vi "Field Mapper.vi"(9 "bandwidth":enum16{"20MHz", "40MHz", "80MHz"}(ring), 10 "subcarrier timing":T2={"subcarrier index"=0, "OFDM symbol index"=0, "frequency offset index"=0.0, "OFDM symbol start"=TRUE, "valid"=TRUE}, 11 "format":enum16{"NON_HT_OFDM", "VHT", "NON_HT_DUP_OFDM"}(ring)) -> (1 "field map":T1, 2 "subcarrier index":fxp<+/-,9,9>)   [LabVIEW 2020]
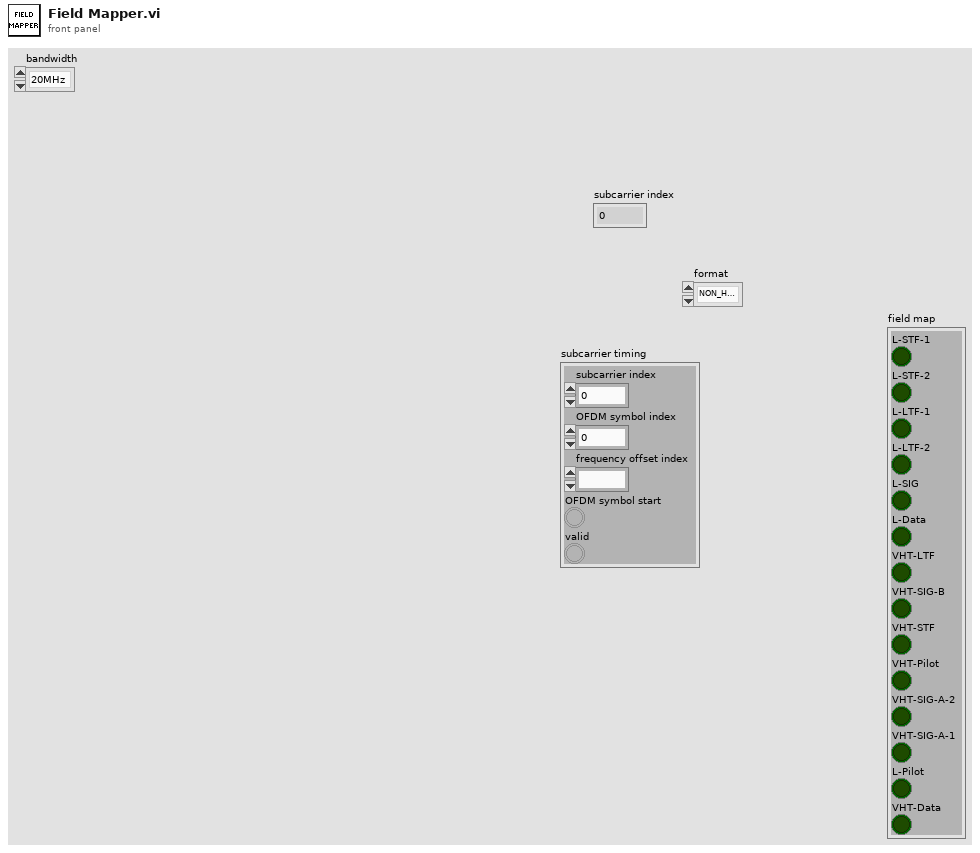
[diagram p1: front panel]
types:
  T1 = cluster{"L-STF-1":bool, "L-STF-2":bool, "L-LTF-1":bool, "L-LTF-2":bool, "L-SIG":bool, "L-Data":bool, "VHT-LTF":bool, "VHT-SIG-B":bool, "VHT-STF":bool, "VHT-Pilot":bool, "VHT-SIG-A-2":bool, "VHT-SIG-A-1":bool, "L-Pilot":bool, "VHT-Data":bool}
  T2 = cluster{"subcarrier index":u8, "OFDM symbol index":u16, "frequency offset index":fxp<+/-,9,9>, "OFDM symbol start":bool, "valid":bool}
  T3 = cluster{"L-STF-1":bool, "L-STF-2":bool, "L-LTF-1":bool, "L-LTF-2":bool, "L-SIG":bool, "VHT-Data":bool, "VHT-Data Init":bool, "VHT-SIG-B":bool, "VHT-LTF":bool, "VHT-STF":bool, "VHT-SIG A-2":bool, "VHT-SIG A-1":bool, "L-Data":bool, "L-Data Init":bool}
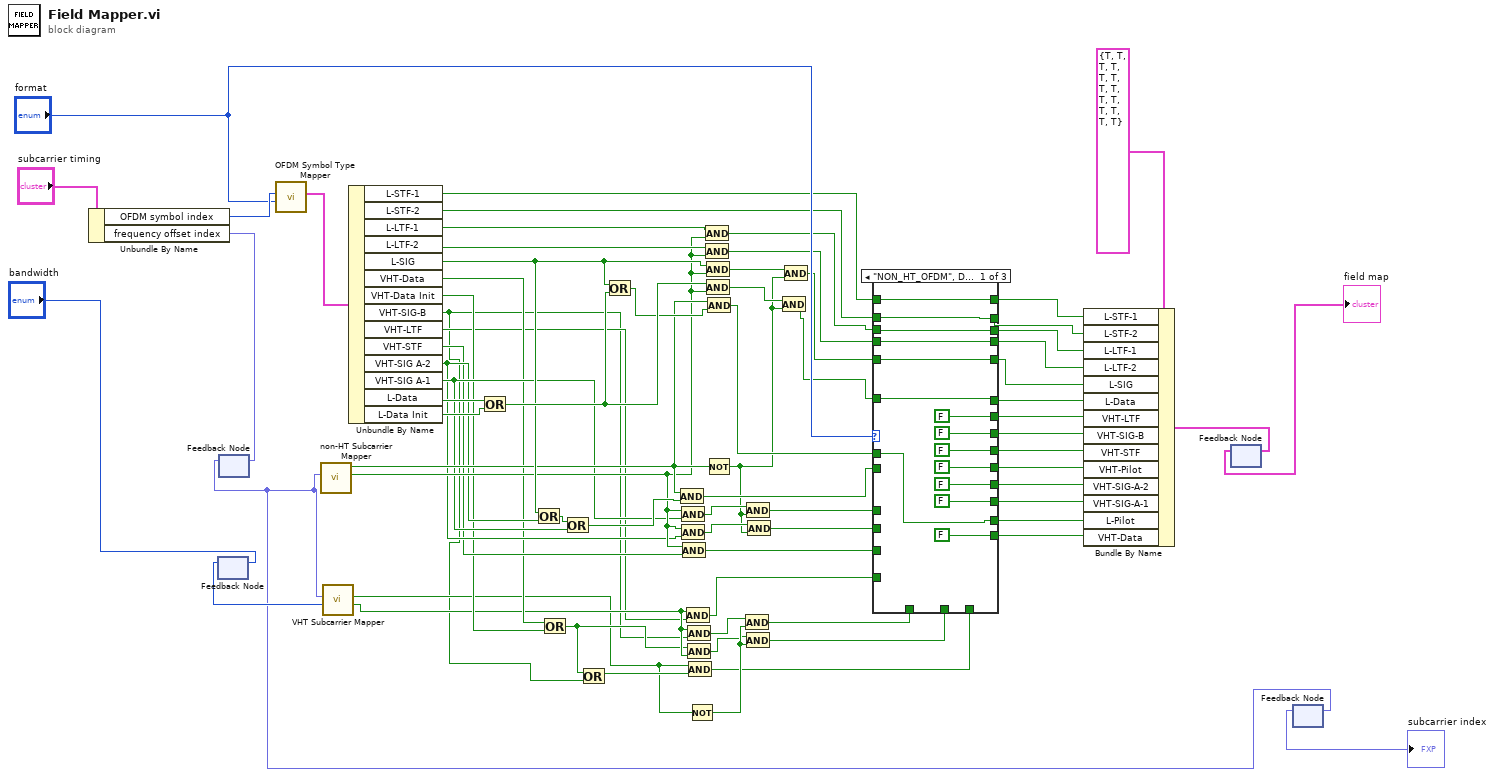
[diagram p0: block diagram]
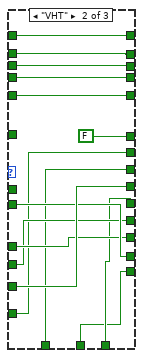
[diagram p2: hidden frame]
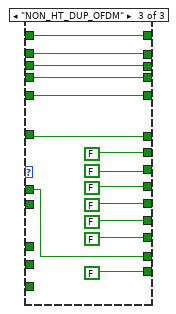
[diagram p3: hidden frame]
diagram:
  n1 = Unbundle By Name("subcarrier timing") -> ("OFDM symbol index"=w70:u16, "frequency offset index"=w68:fxp<+/-,9,9>)
  n2 = feedback #1() -> (w66:enum16{"20MHz", "40MHz", "80MHz"})  [unwired: 1 in]
  n3 = feedback-in #1("bandwidth") -> ()
  n4 = feedback-in #2(w68) -> ()
  n5 = feedback #2() -> (w1:fxp<+/-,9,9>)  [unwired: 1 in]
  n6 = call "OFDM Symbol Type Mapper.vi"("format"="format", "OFDM symbol index"=w70) -> ("Cluster"=w69:T3)  [unwired: 9 in]
  n7 = call "non-HT Subcarrier Mapper.vi"("frequency offset index"=w1) -> ("subcarrier valid"=w30:bool, "pilot subcarrier"=w31:bool)  [unwired: 9 in]
  n8 = call "VHT Subcarrier Mapper.vi"("bandwidth"=w66, "frequency offset index"=w1) -> ("subcarrier valid"=w17:bool, "pilot subcarrier"=w14:bool)  [unwired: 8 in]
  n9 = Unbundle By Name(w69) -> ("L-STF-1"=w54:bool, "L-STF-2"=w52:bool, "L-LTF-1"=w51:bool, "L-LTF-2"=w50:bool, "L-SIG"=w33:bool, "VHT-Data"=w19:bool, "VHT-Data Init"=w18:bool, "VHT-SIG-B"=w5:bool, "VHT-LTF"=w6:bool, "VHT-STF"=w27:bool, "VHT-SIG A-2"=w28:bool, "VHT-SIG A-1"=w29:bool, "L-Data"=w41:bool, "L-Data Init"=w40:bool)
  n10 = Or(x=w41, y=w40) -> (x .or. y?=w38:bool)
  n11 = Or(x=w33, y=w28) -> (x .or. y?=w34:bool)
  n12 = Or(x=w19, y=w18) -> (x .or. y?=w15:bool)
  n13 = Or(x=w34, y=w29) -> (x .or. y?=w32:bool)
  n14 = Or(x=w15, y=w5) -> (x .or. y?=w16:bool)
  n15 = Or(x=w33, y=w38) -> (x .or. y?=w37:bool)
  n16 = And(x=w31, y=w32) -> (x .and. y?=w25:bool)
  n17 = And(x=w30, y=w29) -> (x .and. y?=w24:bool)
  n18 = And(x=w30, y=w28) -> (x .and. y?=w23:bool)
  n19 = And(x=w30, y=w27) -> (x .and. y?=w26:bool)
  n20 = And(x=w17, y=w6) -> (x .and. y?=w7:bool)
  n21 = And(x=w17, y=w5) -> (x .and. y?=w12:bool)
  n22 = And(x=w15, y=w17) -> (x .and. y?=w11:bool)
  n23 = And(x=w14, y=w16) -> (x .and. y?=w10:bool)
  n24 = Not(x=w14) -> (.not. x?=w13:bool)
  n25 = And(x=w51, y=w30) -> (x .and. y?=w48:bool)
  n26 = And(x=w50, y=w30) -> (x .and. y?=w47:bool)
  n27 = And(x=w33, y=w30) -> (x .and. y?=w49:bool)
  n28 = And(x=w38, y=w30) -> (x .and. y?=w42:bool)
  n29 = And(x=w31, y=w37) -> (x .and. y?=w36:bool)
  n30 = Not(x=w31) -> (.not. x?=w22:bool)
  n31 = And(x=w12, y=w13) -> (x .and. y?=w8:bool)
  n32 = And(x=w24, y=w22) -> (x .and. y?=w21:bool)
  n33 = And(x=w11, y=w13) -> (x .and. y?=w9:bool)
  n34 = And(x=w23, y=w22) -> (x .and. y?=w20:bool)
  n35 = And(x=w42, y=w22) -> (x .and. y?=w39:bool)
  n36 = And(x=w49, y=w22) -> (x .and. y?=w46:bool)
  n37 = case shown="\"NON_HT_OFDM\", Default" "format" {
    tunnel: [FALSE ("VHT-SIG-A-1") w91 FALSE ("VHT-SIG-A-1")] -> w63
    tunnel: [FALSE ("VHT-SIG-A-2") w90 FALSE ("VHT-SIG-A-2")] -> w62
    tunnel: [FALSE ("VHT-STF") w93 FALSE ("VHT-STF")] -> w61
    tunnel: [FALSE ("VHT-LTF") w86 FALSE ("VHT-LTF")] -> w60
    tunnel: [FALSE ("VHT-SIG-B") w87 FALSE ("VHT-SIG-B")] -> w59
    tunnel: [FALSE ("VHT-Data") w88 FALSE ("VHT-Data")] -> w58
    tunnel: [FALSE ("VHT-Pilot") w89 FALSE ("VHT-Pilot")] -> w57
    tunnel: [w73 FALSE ("L-Data") w101] -> w56
    tunnel: [w78 w98 w106] -> w55
    tunnel: w54 -> [w78 w98 w106]
    tunnel: [w77 w97 w105] -> w53
    tunnel: w52 -> [w77 w97 w105]
    tunnel: w48 -> [w76 w94 w104]
    tunnel: w47 -> [w75 w95 w103]
    tunnel: w46 -> [w74 w96 w102]
    tunnel: [w76 w94 w104] -> w45
    tunnel: [w75 w95 w103] -> w44
    tunnel: [w74 w96 w102] -> w43
    tunnel: w39 -> [w73 _ w101]
    tunnel: w36 -> [w72 _ w100]
    tunnel: [w72 w92 w100] -> w35
    tunnel: w26 -> [_ w93 _]
    tunnel: w25 -> [_ w92 _]
    tunnel: w21 -> [_ w91 _]
    tunnel: w20 -> [_ w90 _]
    tunnel: w10 -> [_ w89 _]
    tunnel: w9 -> [_ w88 _]
    tunnel: w8 -> [_ w87 _]
    tunnel: w7 -> [_ w86 _]
    frame "NON_HT_OFDM", Default {
    }
    frame "VHT" {
    }
    frame "NON_HT_DUP_OFDM" {
    }
  }
  n38 = Bundle By Name(cluster=T1 {"L-STF-1"=TRUE, "L-STF-2"=TRUE, "L-LTF-1"=TRUE, "L-LTF-2"=TRUE, "L-SIG"=TRUE, "L-Data"=TRUE, "VHT-LTF"=TRUE, "VHT-SIG-B"=TRUE, "VHT-STF"=TRUE, "VHT-Pilot"=TRUE, "VHT-SIG-A-2"=TRUE, "VHT-SIG-A-1"=TRUE, "L-Pilot"=TRUE, "VHT-Data"=TRUE}, "L-STF-1"=w55, "L-STF-2"=w53, "L-LTF-1"=w45, "L-LTF-2"=w44, "L-SIG"=w43, "L-Data"=w56, "VHT-LTF"=w60, "VHT-SIG-B"=w59, "VHT-STF"=w61, "VHT-Pilot"=w57, "VHT-SIG-A-2"=w62, "VHT-SIG-A-1"=w63, "L-Pilot"=w35, "VHT-Data"=w58) -> (w4:T1)
  n39 = feedback-in #3(w4) -> ()
  n40 = feedback #3() -> (→"field map":T1)  [unwired: 1 in]
  n41 = feedback #4() -> (→"subcarrier index":fxp<+/-,9,9>)  [unwired: 1 in]
  n42 = feedback-in #4(w1) -> ()
